vi "UpdateRingsFromDatabase.vi"(8 "error in (no error)":errorcluster, 9 "device":string, 10 "VariablesNames[]":string[](array[string]), 11 "RingsRefs[]":refnum<vi>[](array[refnum])) -> (0 "error out":errorcluster)   [LabVIEW 2013]
doc: "Update the ring indicators"
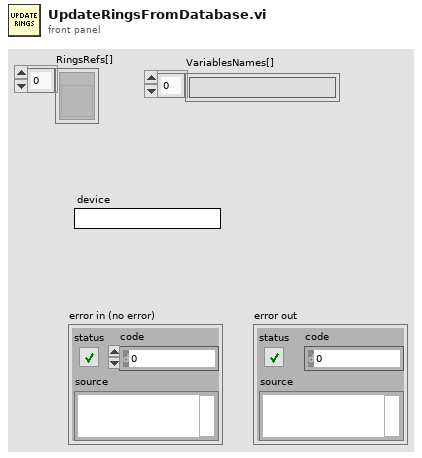
[diagram p1: front panel]
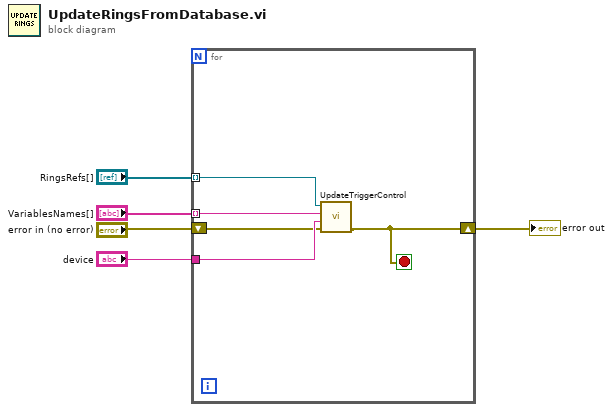
[diagram p0: block diagram]
diagram:
  n1 = for {
    tunnel: "device" -> [w10]
    shift-right: [w6] -> w3
    shift-left: "error in (no error)" -> [w9]
    tunnel: "RingsRefs[]" -> [w8] mode=indexing
    tunnel: "VariablesNames[]" -> [w7] mode=indexing
    stop <- w6 stop-if-true
    n2 = call "UpdateTriggerControl.vi"("error in (no error)"=w9, "Device"=w10, "Varialbe"=w7, "RingRef"=w8) -> ("error IO"=w6:errorcluster)  [unwired: 7 in]
  }
  "error out" <- w3
